vi "SineWaveGenerato.vi"(6 "amplitude":dbl, 7 "Sampling Period":dbl, 8 "Noise Std":dbl=1.0 format="%0.2f", 9 "phase":dbl, 10 "frequency":dbl, 11 "Number of Samples":i32) -> (3 "Array":dbl[](array[numeric]))   [LabVIEW 2019]
uses:
  <vilib>/ptbypt/NI_PtbyPt.lvlib
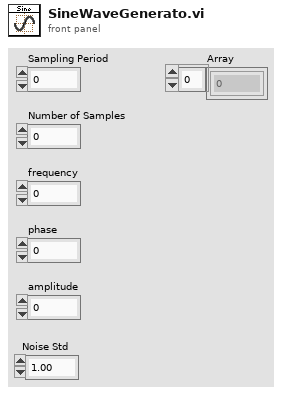
[diagram p1: front panel]
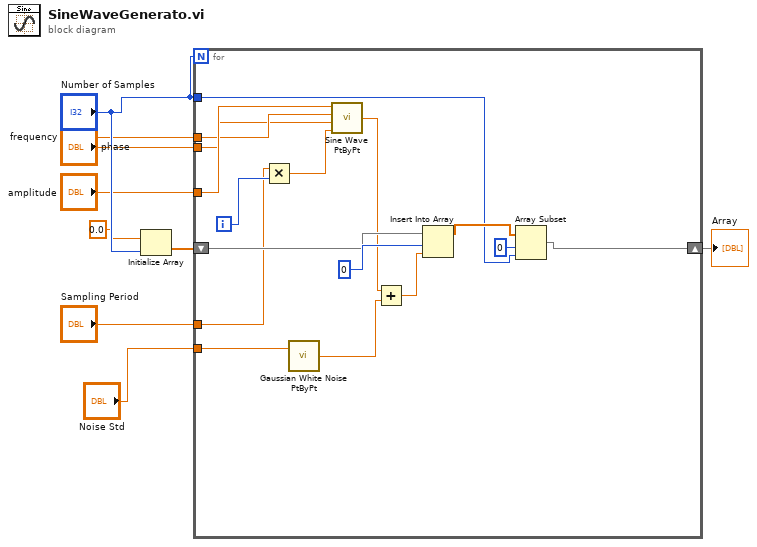
[diagram p0: block diagram]
diagram:
  n1 = Initialize Array(0.0 ("element"), "Number of Samples") -> (w5:dbl[])
  n2 = for {
    N: "Number of Samples" -> [_]
    tunnel: "amplitude" -> [w25]
    tunnel: "frequency" -> [w24]
    tunnel: "phase" -> [w23]
    shift-right: [w14] -> w9
    shift-left: w5 -> [w21]
    tunnel: "Sampling Period" -> [w18]
    tunnel: "Number of Samples" -> [w15]
    tunnel: "Noise Std" -> [w10]
    i -> [w19]
    n3 = Multiply(x=w18, y=w19) -> (x*y=w20:dbl)
    n4 = call <vilib>:"Gaussian White Noise PtByPt.vi"("standard deviation"=w10) -> ("Gaussian white noise"=w12:dbl)  [unwired: 2 in]
    n5 = call <vilib>:"Sine Wave PtByPt.vi"("time"=w20, "phase"=w23, "frequency"=w24, "amplitude"=w25) -> ("sine wave"=w13:dbl)
    n6 = Add(x=w13, y=w12) -> (x+y=w11:dbl)
    n7 = Insert Into Array(array=w21, index=0, new element=w11) -> (w17:dbl[])
    n8 = Array Subset(array=w17, index=0, length=w15) -> (w14:dbl[])
  }
  "Array" <- w9
